vi "Формула_1.vi"() -> ()   [LabVIEW 2020]
panel:
  out "Numer":dbl
  in  "X":dbl
  # "X^2 - sin(5*X) ="
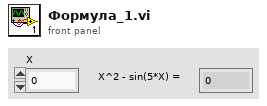
[diagram p1: front panel]
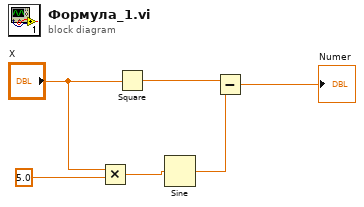
[diagram p0: block diagram]
diagram:
  n1 = Multiply(x="X", y=5.0 ("a")) -> (x*y=w3:dbl)
  n2 = Square(x="X") -> (x^2=w6:dbl)
  n3 = Sine(x=w3) -> (sin(x)=w2:dbl)
  n4 = Subtract(x=w6, y=w2) -> (x-y=→"Numer":dbl)
